vi "Voltage_file.vi"() -> ()   [LabVIEW 2010]
uses:
  <vilib>/Utility/file.llb/Read From Spreadsheet File (DBL).vi
  <vilib>/Utility/file.llb/Write To Spreadsheet File (DBL).vi
  <instrlib>/lib-labview-8.6-export/Keithley-6482-Visa.lvlib
panel:
  out "Voltage table":dbl[][](array[numeric])
  in  "Error In":errorcluster
  out "V2":dbl[](array[numeric])
  out "V1":dbl[](array[numeric])
  in  "xoffset":u16=1
  in  "width":u16=1340
  in  "xbin":u16=1
  in  "Integrations":i32=1
  in  "yoffset":u16=1
  in  "height":u16=100
  in  "ybin":u16=1
  in  "Center wavelength":dbl=650.0
  in  "Grating":bool=TRUE
  in  "Exposure time (s)":dbl=0.1 format="%.2f"
  out "XY Graph":cluster{dbl[], dbl[]}(graph) caption="Spectrum"
  in  "File name":string="HT78_300G_650C_0.1s_100int_15swait"
  in  "initial wait (ms)":dbl=300000.0
  in  "wait time (ms)`":dbl=15000.0
  out "Current V1":dbl
  out "Current":dbl[](array[numeric])
  out "Current V2":dbl
  in  "Voltage file":path=path "C:/Users/Pump probe_B145/Desktop/data/Delay/Delay_longscan_6t0_linarray_2.txt"
  out "Error Out":errorcluster
  in  "base path":path=path "C:/Users/Pump probe_B145/Desktop/data/2019/190630/gate_abs/GBG_N1V_GBG_2VtoN2V_GBGregion"
  in  "VISA resource name":refnum<visa-resource-name>="GPIB0::20::INSTR"
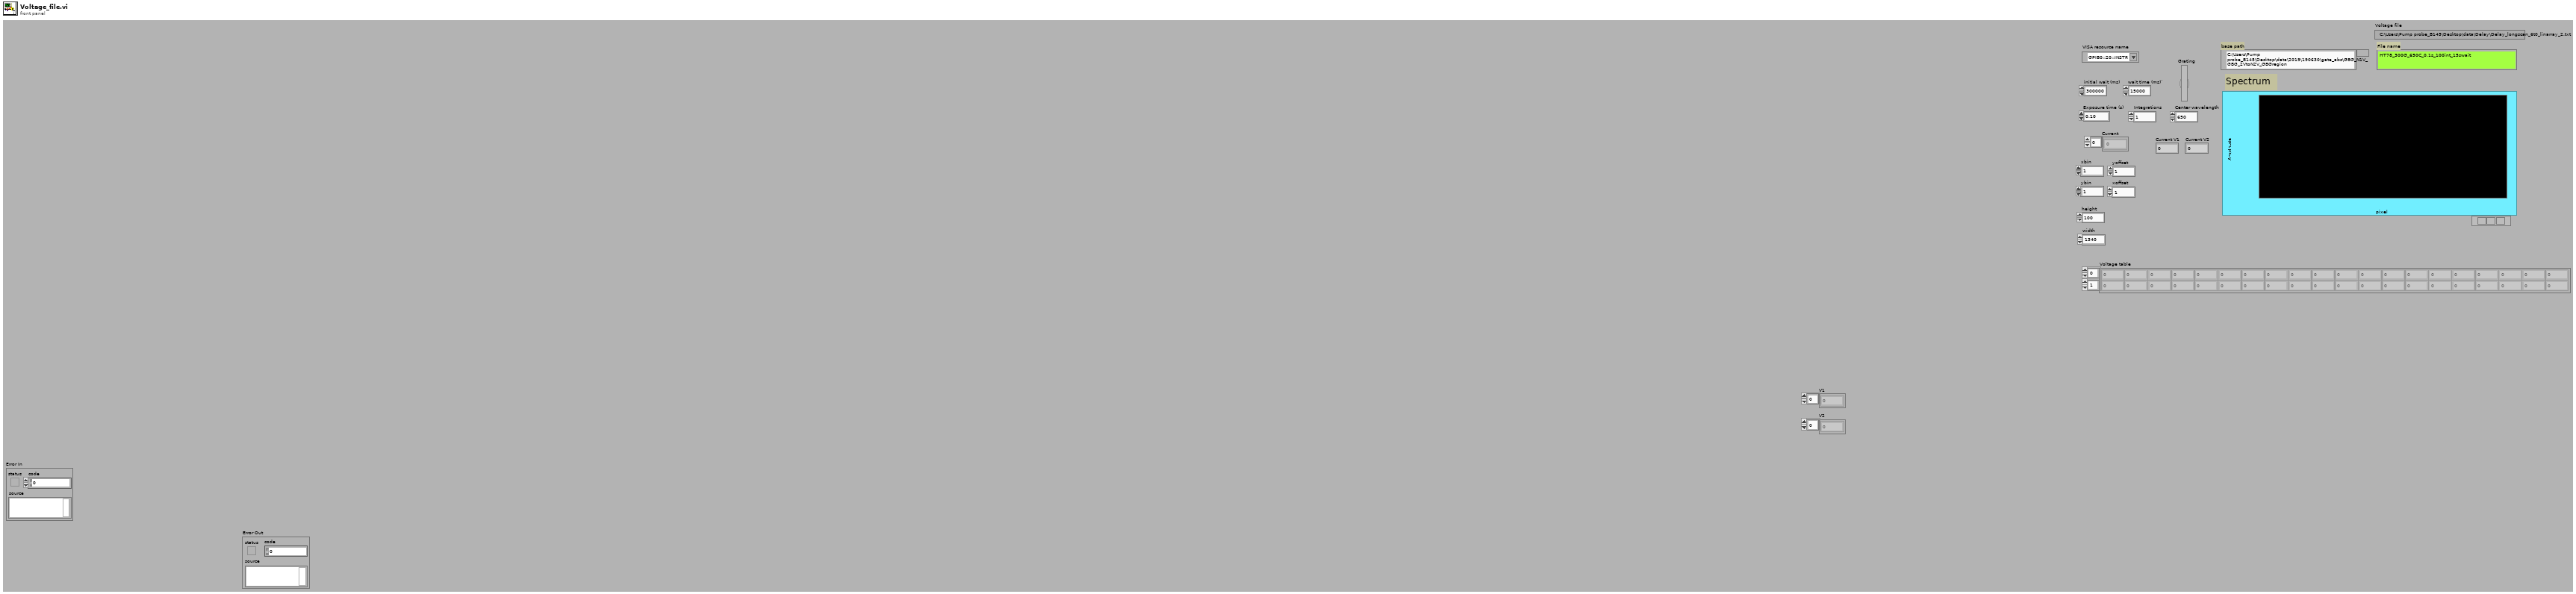
[diagram p1: front panel]
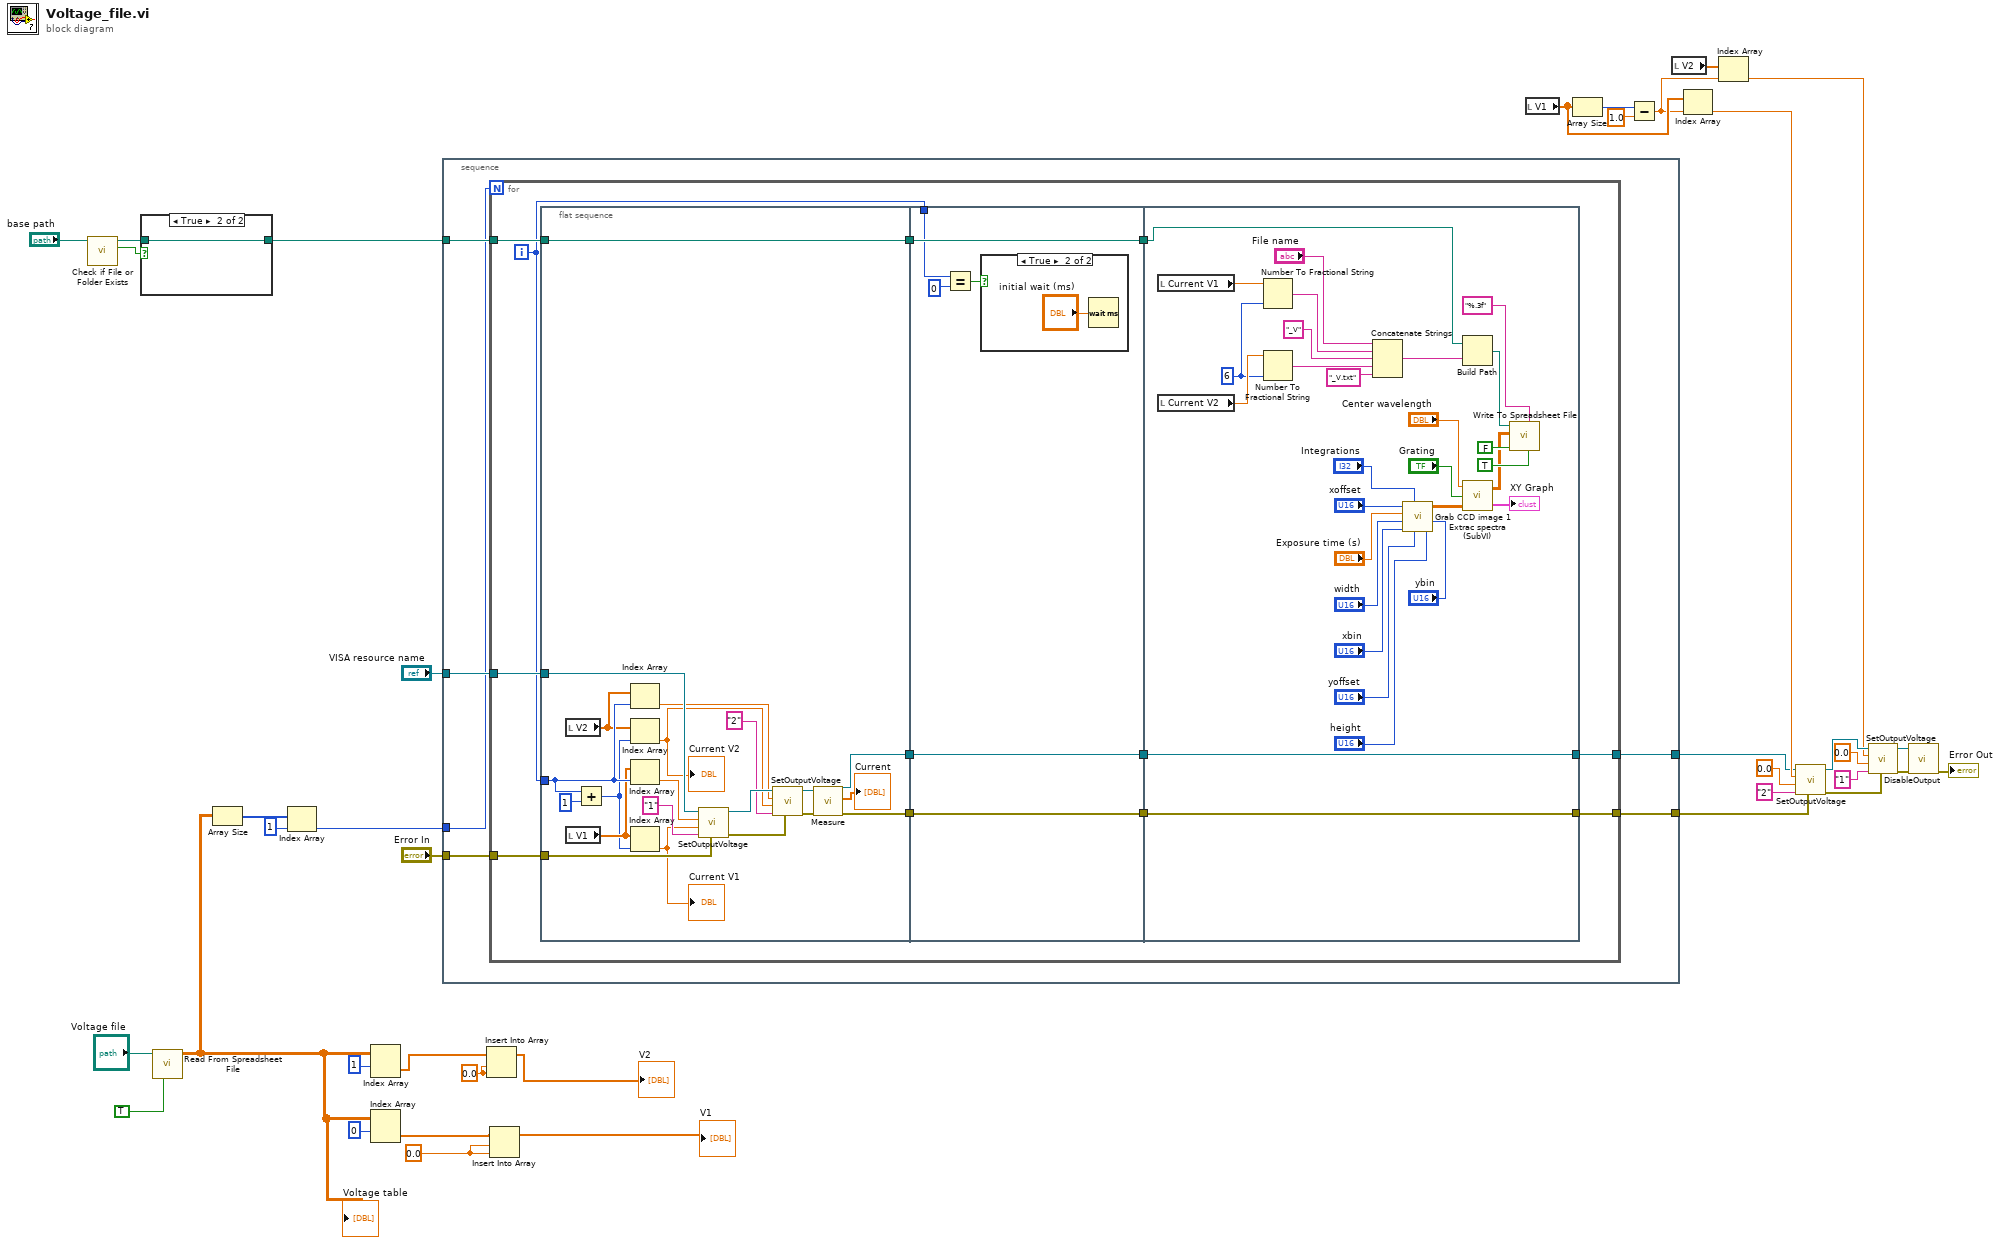
[diagram p0: block diagram]
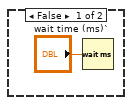
[diagram p2: hidden frame]
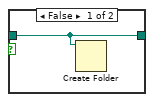
[diagram p3: hidden frame]
diagram:
  w1 = 0.0 ("new element/subarray")
  w2 = 0.0 ("new element/subarray")
  n1 = call <vilib>:"Check if File or Folder Exists.vi"("path"="base path") -> ("file or folder exists?"=w37:bool, "dup path"=w38:path)  [unwired: 8 in, 1 out]
  n2 = case shown="True" w37 {
    tunnel: w38 -> [w39 w40]
    tunnel: [w39 w40] -> w35
    frame False {
      n3 = Create Folder(path (use dialog)=w39) -> ()  [unwired: 2 in, 3 out]
    }
    frame True {
    }
  }
  n4 = call-poly <vilib>:"Read From Spreadsheet File.vi"("transpose (no:F)"=TRUE, "file path (dialog if empty)"="Voltage file") -> ("all rows"=w8:dbl[][])  [unwired: 5 in, 4 out]
  "Voltage table" <- w8
  n5 = Array Size(array=w8) -> (size(s)=w21:i32[])
  n6 = Index Array(array=w21, index=1) -> (element=w3:i32)
  n7 = Index Array(array=w8, index (row)=1) -> (element=w7:dbl[])  [unwired: 1 in]
  n8 = Index Array(array=w8, index (row)=0) -> (element=w5:dbl[])  [unwired: 1 in]
  n9 = stacked-sequence {
    tunnel: "VISA resource name" -> [w43]
    tunnel: w35 -> [w46]
    tunnel: [w45] -> w10
    tunnel: [w44] -> w9
    tunnel: "Error In" -> [w42]
    tunnel: w3 -> [w41]
    frame #0 {
      n10 = for {
        N: w41 -> [_]
        tunnel: w43 -> [w58]
        tunnel: w46 -> [w57]
        tunnel: [w52] -> w45
        tunnel: [w50] -> w44
        tunnel: w42 -> [w48]
        i -> [w47]
        n11 = flat-sequence {
          tunnel: w58 -> [w78]
          tunnel: [w79] -> w56
          tunnel: w57 -> [w79]
          tunnel: [w76] -> w53
          tunnel: [w75] -> w49
          tunnel: w48 -> [w77]
          tunnel: w47 -> [w65]
          tunnel: w56 -> [w85]
          tunnel: [w85] -> w55
          tunnel: w47 -> [w84]
          tunnel: [w81] -> w54
          tunnel: w53 -> [w81]
          tunnel: [w80] -> w51
          tunnel: w49 -> [w80]
          tunnel: w55 -> [w97]
          tunnel: w54 -> [w96]
          tunnel: [w96] -> w52
          tunnel: w51 -> [w95]
          tunnel: [w95] -> w50
          frame #0 {
            n12 = local read "V2"() -> (w61:dbl[])
            n13 = local read "V1"() -> (w63:dbl[])
            n14 = Add(x=w65, y=1) -> (x+y=w60:i32)
            n15 = Index Array(array=w61, index=w65) -> (element=w66:dbl)
            n16 = Index Array(array=w61, index=w60) -> (element=w59:dbl)
            "Current V2" <- w59
            n17 = Index Array(array=w63, index=w65) -> (element=w72:dbl)
            n18 = Index Array(array=w63, index=w60) -> (element=w62:dbl)
            "Current V1" <- w62
            n19 = call <instrlib>:"SetOutputVoltage.vi"("Error In"=w77, "channel(1,2)"="1", "Voltage"=w62, "V_pre"=w72, "Keithley 6482"=w78) -> ("Error Out"=w69:errorcluster, "Keithley 6483"=w71:refnum<visa-resource-name>)  [unwired: 5 in]
            n20 = call <instrlib>:"SetOutputVoltage.vi"("Error In"=w69, "channel(1,2)"="2", "Voltage"=w59, "V_pre"=w66, "Keithley 6482"=w71) -> ("Error Out"=w68:errorcluster, "Keithley 6483"=w70:refnum<visa-resource-name>)  [unwired: 5 in]
            n21 = call <instrlib>:"Measure.vi"("Error In"=w68, "Keithley 6482 In"=w70) -> ("Error Out"=w75:errorcluster, "Values"=→"Current":dbl[], "Keithley 6482 Out"=w76:refnum<visa-resource-name>)  [unwired: 7 in]
          }
          frame #1 {
            n22 = Equal?(x=w84, y=0) -> (x = y?=w83:bool)
            n23 = case shown="True" w83 {
              frame False {
                n24 = Wait (ms)(milliseconds to wait="wait time (ms)`") -> ()  [unwired: 1 out]
              }
              frame True {
                n25 = Wait (ms)(milliseconds to wait="initial wait (ms)") -> ()  [unwired: 1 out]
              }
            }
          }
          frame #2 {
            w91 = 6
            n26 = local read "Current V1"() -> (w93:dbl)
            n27 = local read "Current V2"() -> (w92:dbl)
            n28 = Number To Fractional String(number=w93, precision (6)=w91) -> (F-format string=w89:string)  [unwired: 2 in]
            n29 = Number To Fractional String(number=w92, precision (6)=w91) -> (F-format string=w90:string)  [unwired: 2 in]
            n30 = Concatenate Strings("File name", w89, "_V" ("string"), w90, "_V.txt" ("Substring")) -> (w99:string)
            n31 = call "Grab CCD image 1.vi"("height"="height", "ybin"="ybin", "yoffset"="yoffset", "Average time"="Integrations", "xbin"="xbin", "width"="width", "Exposure time (s)"="Exposure time (s)", "xoffset"="xoffset") -> ("CCD image"=w108:dbl[][])  [unwired: 1 out]
            n32 = Build Path(base path=w97, name or relative path=w99) -> (appended path=w98:path)
            n33 = call "Extrac spectra (SubVI).vi"("CCD image"=w108, "Grating (1:300nm/0:1200nm)"="Grating", "Center wavelength"="Center wavelength") -> ("XY Graph"=→"XY Graph":cluster{dbl[], dbl[]}, "appended array"=w101:dbl[][])
            n34 = call-poly <vilib>:"Write To Spreadsheet File.vi"("transpose? (no:F)"=TRUE, "format (%.3f)"="%.3f", "append to file? (new file:F)"=FALSE, "2D data"=w101, "file path (dialog if empty)"=w98) -> ()  [unwired: 3 in, 1 out]
          }
        }
      }
    }
  }
  n35 = Insert Into Array(array=w7, index=w2, new element=w2) -> (→"V2":dbl[])
  n36 = Insert Into Array(array=w5, index=w1, new element=w1) -> (→"V1":dbl[])
  n37 = local read "V1"() -> (w17:dbl[])
  n38 = Array Size(array=w17) -> (size(s)=w12:i32)
  n39 = Subtract(x=w12, y=1.0) -> (x-y=w11:dbl)
  n40 = local read "V2"() -> (w16:dbl[])
  n41 = Index Array(array=w17, index=w11) -> (element=w14:dbl)
  n42 = Index Array(array=w16, index=w11) -> (element=w15:dbl)
  n43 = call <instrlib>:"SetOutputVoltage.vi"("Error In"=w9, "channel(1,2)"="2", "Voltage"=0.0, "V_pre"=w14, "Keithley 6482"=w10) -> ("Error Out"=w26:errorcluster, "Keithley 6483"=w30:refnum<visa-resource-name>)  [unwired: 5 in]
  n44 = call <instrlib>:"SetOutputVoltage.vi"("Error In"=w26, "channel(1,2)"="1", "Voltage"=0.0, "V_pre"=w15, "Keithley 6482"=w30) -> ("Error Out"=w28:errorcluster, "Keithley 6483"=w29:refnum<visa-resource-name>)  [unwired: 5 in]
  n45 = call <instrlib>:"DisableOutput.vi"("Error In"=w28, "Keithley 6482 In"=w29) -> ("Error Out"=→"Error Out":errorcluster)  [unwired: 8 in, 1 out]
